vi "Configure Trigger.vi"(7 "Trigger Type":u16(ring) items=["Bus", "Manual"], 8 "error in (no error)":errorcluster, 9 "Trigger Current Limit (0.0 A)":dbl format="%.2g", 10 "Trigger Voltage Limit (0.0 V)":dbl format="%.2g", 11 "VISA resource name":refnum<visa-resource-name>) -> (0 "error out":errorcluster, 3 "VISA resource name out":refnum<visa-resource-name>)   [LabVIEW 2013, in "IT6900.lvlib"]
doc: "This command is used to select the source of the trigger signal. The power source can receive a trigger signal from the panel (keyboard trigger Trigger key) or receive the bus trigger signal.\nAnd set the limit voltage and current."
uses:
  IT6900.lvlib
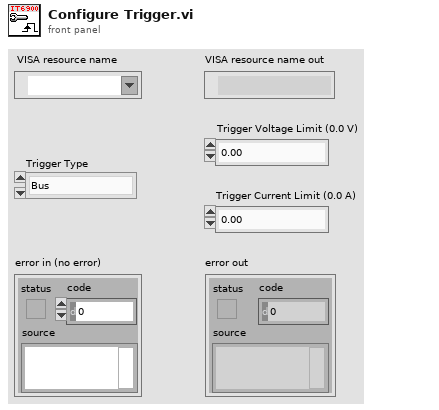
[diagram p1: front panel]
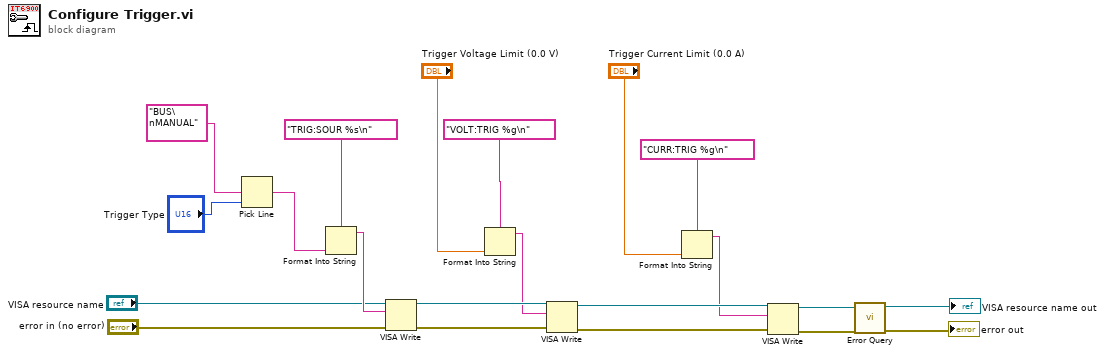
[diagram p0: block diagram]
diagram:
  n1 = Pick Line(multi-line string="BUS\nMANUAL", line index="Trigger Type") -> (output string=w19:string)  [unwired: 1 in]
  n2 = Format Into String(format string="TRIG:SOUR %s\n", w19) -> (resulting string=w13:string)  [unwired: 2 in, 1 out]
  n3 = VISA Write(VISA resource name="VISA resource name", write buffer=w13, error in (no error)="error in (no error)") -> (VISA resource name out=w10:refnum<visa-resource-name>, error out=w9:errorcluster)  [unwired: 1 out]
  n4 = Format Into String(format string="VOLT:TRIG %g\n", "Trigger Voltage Limit (0.0 V)") -> (resulting string=w6:string)  [unwired: 2 in, 1 out]
  n5 = VISA Write(VISA resource name=w10, write buffer=w6, error in (no error)=w9) -> (VISA resource name out=w8:refnum<visa-resource-name>, error out=w7:errorcluster)  [unwired: 1 out]
  n6 = Format Into String(format string="CURR:TRIG %g\n", "Trigger Current Limit (0.0 A)") -> (resulting string=w5:string)  [unwired: 2 in, 1 out]
  n7 = VISA Write(VISA resource name=w8, write buffer=w5, error in (no error)=w7) -> (VISA resource name out=w3:refnum<visa-resource-name>, error out=w4:errorcluster)  [unwired: 1 out]
  n8 = call "Error Query.vi"("error in (no error)"=w4, "VISA resource name"=w3) -> ("error out"=→"error out":errorcluster, "VISA resource name out"=→"VISA resource name out":refnum<visa-resource-name>)  [unwired: 6 in, 2 out]
